vi "Step_SetHiSpeed.vi"(7 "HiSpeed":dbl, 8 "error in (no error)":errorcluster, 10 "device_reference":i32, 11 "WindmillDevice in":refnum<class "WindmillDevice.lvclass">) -> (0 "error out":errorcluster, 3 "WindmillDevice out":refnum<class "WindmillDevice.lvclass">)   [LabVIEW 2020, in "WindmillDevice.lvclass"]
uses:
  WindmillDevice.lvclass
  WindmillDevice.lvclass/WindmillDevice.ctl
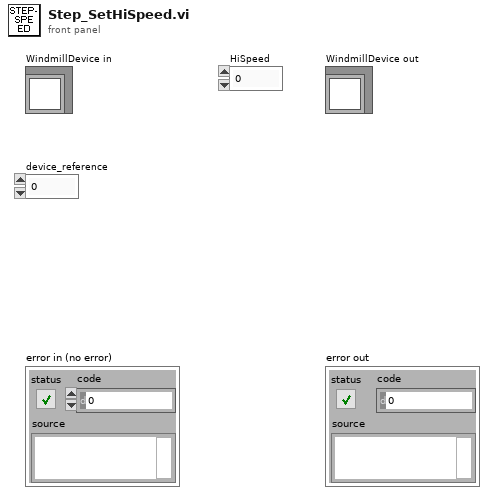
[diagram p1: front panel]
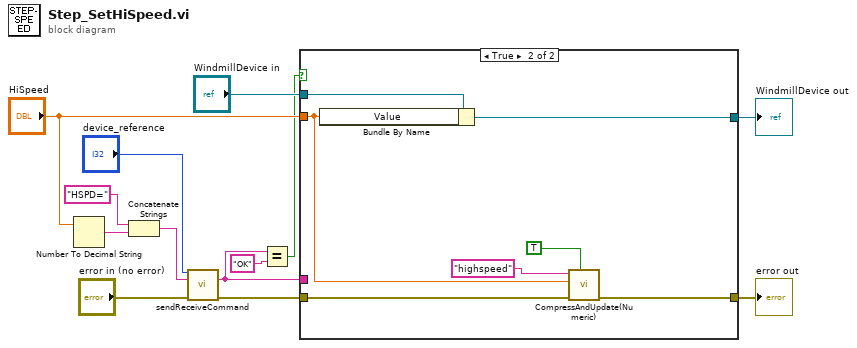
[diagram p0: block diagram]
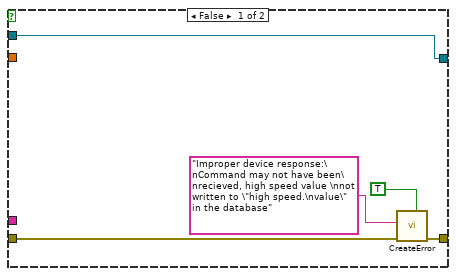
[diagram p2: hidden frame]
diagram:
  n1 = Number To Decimal String(number="HiSpeed") -> (decimal integer string=w13:string)  [unwired: 1 in]
  n2 = Concatenate Strings("HSPD=" ("write_string"), w13) -> (w3:string)
  n3 = call "sendReceiveCommand.vi"("reference (in)"="device_reference", "write_string"=w3, "error in (no error)"="error in (no error)") -> ("read_string"=w9:string, "error out"=w7:errorcluster)  [unwired: 10 in, 1 out]
  n4 = Equal?(x=w9, y="OK") -> (x = y?=w6:bool)
  n5 = case shown="True" w6 {
    tunnel: "HiSpeed" -> [_ w20]
    tunnel: w7 -> [w17 w24]
    tunnel: [w16 w23] -> w8
    tunnel: w9 -> [_ _]
    tunnel: [w18 w22] -> w11
    tunnel: "WindmillDevice in" -> [w18 w21]
    frame False {
      n6 = call "CreateError.vi"("Warning"=TRUE, "user error in"=w17, "error message (\"\")"="Improper device response:\nCommand may not have been\nrecieved, high speed value \nnot written to \"high speed.\nvalue\" in the database" ("error message (\"\")")) -> ("user error  out"=w16:errorcluster)  [unwired: 8 in]
    }
    frame True {
      n7 = Bundle By Name(cluster=w21, "Value"=w20) -> (w22:refnum<class "WindmillDevice.lvclass">)
      n8 = call "CompressAndUpdate(Numeric).vi"("force CVT update (false)"=TRUE, "error in"=w24, "Numeric"=w20, "command or variable name"="highspeed") -> ("error out"=w23:errorcluster)  [unwired: 7 in]
    }
  }
  "WindmillDevice out" <- w11
  "error out" <- w8
